vi "PRO_Check_ResistorLogicV1.vi"(10 "Inputs":cluster{" Ohms":dbl, "Level OUt":dbl}={" Ohms"=101.0, "Level OUt"=7.735}, 11 "ChA Spec RNG In":T2={"Specs"=[7.46, 7.56, 7.91, 202.0, 198.0, 102.0, 98.0], "LUT Status"={"ChA/!ChB"=TRUE, "Drain/!Fill"=FALSE, "In Range?"=TRUE, "Switch Range?"=FALSE, "Measure R?"=FALSE, "Vaild R?"=TRUE, "Index(n)"=2, "Index(n-1)"=1, "Index Max"=13}}) -> (0 "Vaild R?":bool=TRUE, 1 "LUT Status":T1={"ChA/!ChB"=TRUE, "Drain/!Fill"=FALSE, "In Range?"=TRUE, "Switch Range?"=FALSE, "Measure R?"=FALSE, "Vaild R?"=TRUE, "Index(n)"=2, "Index(n-1)"=1, "Index Max"=13}, 2 "Resist Measured":dbl=101.0, 3 "Resist Nominal":dbl=100.0, 4 "Resist in Spec":bool=TRUE, 5 "Drain/!Fill":bool)   [LabVIEW 2024]
uses:
  Control Definitions/Def Spec RNG.ctl
  Control Definitions/Ded LUT_Status.ctl
panel:
  out "ChA/!ChB":bool
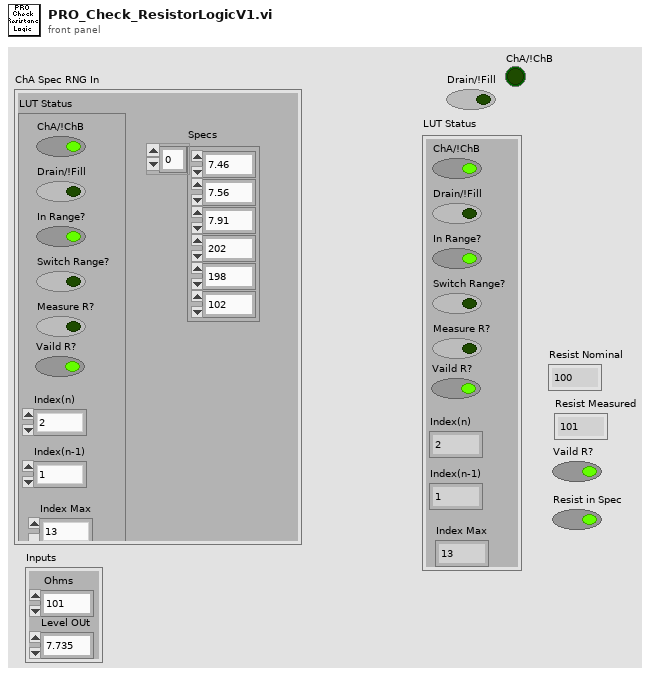
[diagram p1: front panel]
types:
  T1 = typedef "Ded LUT_Status.ctl" = cluster{"ChA/!ChB":bool, "Drain/!Fill":bool, "In Range?":bool, "Switch Range?":bool, "Measure R?":bool, "Vaild R?":bool, "Index(n)":i32, "Index(n-1)":i32, "Index Max":i32}
  T2 = typedef "Def Spec RNG.ctl" = cluster{"Specs":dbl[], "LUT Status":T1}
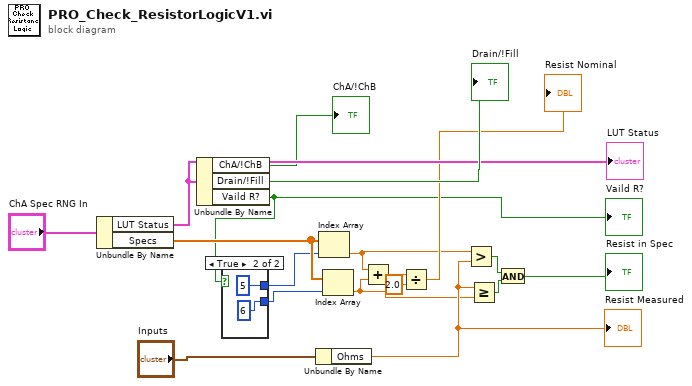
[diagram p0: block diagram]
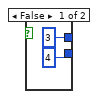
[diagram p2: hidden frame]
diagram:
  n1 = Unbundle By Name("ChA Spec RNG In") -> ("LUT Status"=w15:T1, "Specs"=w5:dbl[])
  "LUT Status" <- w15
  n2 = Unbundle By Name(w15) -> ("ChA/!ChB"=→"ChA/!ChB":bool, "Drain/!Fill"=→"Drain/!Fill":bool, "Vaild R?"=w2:bool)
  "Vaild R?" <- w2
  n3 = case shown="True" w2 {
    tunnel: [3 ("index") 5 ("index")] -> w4
    tunnel: [4 ("index") 6 ("index")] -> w3
    frame False {
    }
    frame True {
    }
  }
  n4 = Unbundle By Name("Inputs") -> ("Ohms"=w13:dbl)
  "Resist Measured" <- w13
  n5 = Index Array(array=w5, index=w4) -> (element=w6:dbl)
  n6 = Index Array(array=w5, index=w3) -> (element=w10:dbl)
  n7 = Add(x=w6, y=w10) -> (x+y=w7:dbl)
  n8 = Divide(x=w7, y=2.0) -> (x/y=→"Resist Nominal":dbl)
  n9 = Greater?(x=w6, y=w13) -> (0:w12:bool)
  n10 = Greater Or Equal?(x=w13, y=w10) -> (x >= y?=w11:bool)
  n11 = And(x=w12, y=w11) -> (x .and. y?=→"Resist in Spec":bool)
